vi "Main_TestStand_v2.vi"() -> ()   [LabVIEW 2019]
uses:
  <vilib>/Platform/TimedLoop/XDataNode/timing_clust.ctl
  <vilib>/Platform/TimedLoop/XDataNode/nitl_modes.ctl
  <vilib>/Platform/TimedLoop/XDataNode/wakeup.ctl
  <vilib>/platform/TimedLoop/XDataNode/XDataNode.xnode
  <vilib>/ptbypt/NI_PtbyPt.lvlib
  <vilib>/Platform/TimedLoop/XDataNode/XDNodeRunTimeDep.lvlib
panel:
  out "motor signal":cluster{dbl, dbl}
  out "raw x axis imu data":i16
  out "motor 1 correction":dbl(graph)
  out "Labview PID Inputs (should not match gains) 2":T1
  in  "Proportional Gain (Kc) 2":dbl
  in  "Derivative Gain (Kd) 2":dbl format="%#_13g"
  in  "Integral Gain (Ki) 2":dbl format="%#_13g"
  out "Raw x value":dbl(graph)
  in  "Adjustment x":dbl format="%0.2f"
  in  "low cutoff freq x":dbl=0.01 format="%#_13g"
  out "Filtered Correction x":dbl format="%0.2f"
  out "Filtered Correction x":dbl(graph)
  out "Motor 2 Correction":dbl
  out "Motor 1 Correction":dbl
  out "error out":errorcluster
  out "error out 2":errorcluster
  out "error out 6":errorcluster
  in  "Initial Motor Power":dbl
  in  "Stop":bool
  # "X-Axis Gains"
  # "Y-Axis Gains"
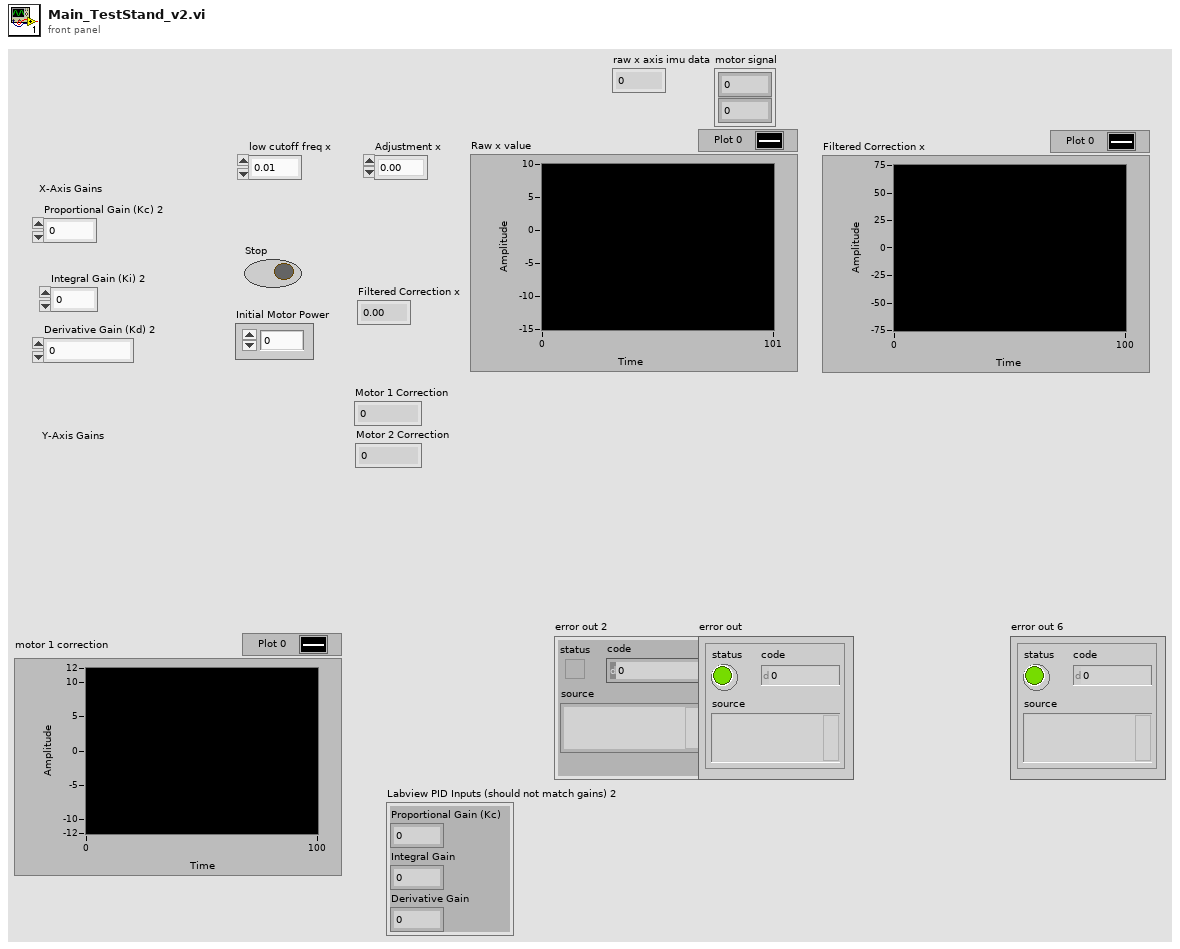
[diagram p1: front panel]
types:
  T1 = cluster{"Proportional Gain (Kc)":dbl, "Integral Gain":dbl, "Derivative Gain":dbl}
  T2 = typedef "XDNodeRunTimeDep.lvlib/timing_clust.ctl" = cluster{"Expected End [f-1]":u64, "Actual End [f-1]":u64, "Finished Late? [f-1]":bool, "Expected End [i-1]":u64, "Actual End [i-1]":u64, "Finished Late? [i-1]":bool, "Expected Start [i]":u64, "Actual Start [i]":u64, "Expected Start [f]":u64, "Actual Start [f]":u64, "Source Name":string, "Structure Name":string, "Period":i64, "Deadline":i64, "Offset":i64, "Start":i64, "Priority":i32, "Timeout":i32, "Mode":T3, "Wakeup Reason":T4, "Error":errorcluster, "Source Type":string, "Secondary Source Type":string, "Global End Time":u64, "Global Start Time":u64, "Frame Duration":u64, "Iteration Duration":u64, "Assigned CPU":i32, "I/O Scan Engine Mode":u32}
  T3 = typedef "XDNodeRunTimeDep.lvlib/nitl_modes.ctl" = enum32{"No Change", "Process missed periods, maintain original phase", "Discard missed periods, maintain original phase", "Process missed periods, ignore original phase", "Discard missed periods, ignore original phase"}
  T4 = typedef "XDNodeRunTimeDep.lvlib/wakeup.ctl" = enum32{"Normal", "Aborted", "Asynchronous wakeup", "Timing source error", "Timed loop error", "Timeout"}
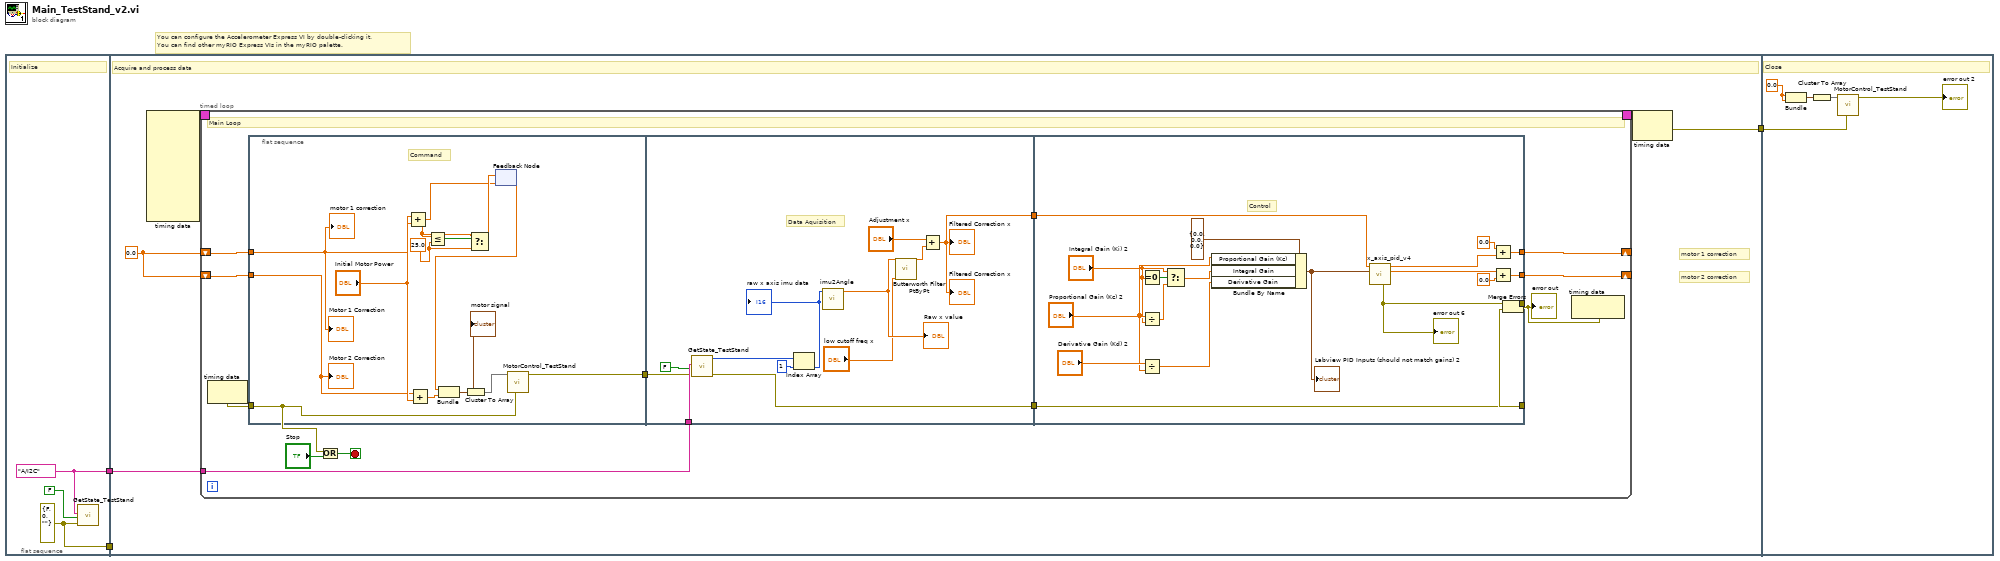
[diagram p0: block diagram]
diagram:
  # "You can configure the Accelerometer Express VI by double-clicking it.\nYou can find other myRIO Express VIs in the myRIO palette."
  n1 = flat-sequence {
    tunnel: [w6] -> w3
    tunnel: [w4] -> w2
    tunnel: [w7] -> w1
    tunnel: w3 -> [w11]
    tunnel: w2 -> [_]
    tunnel: w1 -> [w78]
    frame #0 {
      w6 = tag "A/I2C" ("IMU Channel")
      w4 = errorcluster {"status"=FALSE, "code"=0, "source"=""} ("error in (no error)")
      # "Initialize"
      n2 = call "GetState_TestStand.vi"("error in (no error)"=w4, "Calibrate?"=FALSE, "IMU Channel"=w6) -> ()  [unwired: 4 in, 3 out]
    }
    frame #1 {
      w8 = 0.0
      # "motor 2 correction"
      # "motor 1 correction"
      # "Acquire and process data"
      n3 = node-c288() -> (w10:T2)  [unwired: 9 in]
      n4 = timed-loop {
        tunnel: w11 -> [w22]
        timing: w10 -> [_]
        timing-out: [_] -> w9
        shift-right: [w19] -> _
        shift-left: w8 -> [w17]
        shift-right: [w18] -> _
        shift-left: w8 -> [w16]
        stop <- w25 stop-if-true
        # "Main Loop"
        n5 = node-c288() -> (w12:errorcluster)  [unwired: 1 in]
        n6 = flat-sequence {
          tunnel: w17 -> [w31]
          tunnel: w16 -> [w34]
          tunnel: w12 -> [w33]
          tunnel: [w32] -> w15
          tunnel: w22 -> [w50]
          tunnel: [w41] -> w21
          tunnel: w15 -> [w40]
          tunnel: [w39] -> w14
          tunnel: [w59] -> w23
          tunnel: w21 -> [w58]
          tunnel: [w55] -> w19
          tunnel: [w54] -> w18
          tunnel: w14 -> [w51]
          tunnel: [w51] -> w13
          frame #0 {
            w27 = 25.0 ("y")
            # "Command"
            n7 = Add(x=w31, y="Initial Motor Power") -> (x+y=w26:dbl)
            n8 = Add(x=w34, y="Initial Motor Power") -> (x+y=w38:dbl)
            n9 = Less Or Equal?(x=w26, y=w27) -> (x <= y?=w28:bool)
            n10 = Select(t=w26, s=w28, f=w27) -> (s? t:f=w30:dbl)
            n11 = feedback-in #1(w30) -> ()
            n12 = feedback #1(w26) -> (w29:dbl)
            n13 = Bundle(w29, w38) -> (w36:cluster{dbl, dbl})  [unwired: 1 in]
            "motor signal" <- w36
            n14 = Cluster To Array(cluster=w36) -> (array=w35:dbl[])
            n15 = call "MotorControl_TestStand.vi"("error in (no error)"=w33, "Array"=w35) -> ("error out"=w32:errorcluster)  [unwired: 9 in]
            "Motor 1 Correction" <- w31
            "Motor 2 Correction" <- w34
            "motor 1 correction" <- w31
          }
          frame #1 {
            # "Data Aquisition"
            n16 = call "GetState_TestStand.vi"("error in (no error)"=w40, "Calibrate?"=FALSE, "IMU Channel"=w50) -> ("error out"=w39:errorcluster, "imu accel"=w43:i16[])  [unwired: 4 in, 1 out]
            n17 = Index Array(array=w43, index=1) -> (element=w42:i16)
            "raw x axis imu data" <- w42
            n18 = call "imu2Angle.vi"("Sensor Input"=w42) -> ("Angle (radians)"=w48:dbl)  [unwired: 10 in]
            "Raw x value" <- w48
            n19 = call <vilib>:"Butterworth Filter PtByPt.vi"("low cutoff freq: fl"="low cutoff freq x", "x"=w48) -> ("Filtered x"=w46:dbl)  [unwired: 7 in, 1 out]
            n20 = Add(x="Adjustment x", y=w46) -> (x+y=w41:dbl)
            "Filtered Correction x" <- w41
            "Filtered Correction x" <- w41
          }
          frame #2 {
            # "Control"
            n21 = Equal To 0?(x="Integral Gain (Ki) 2") -> (x = 0?=w64:bool)
            n22 = Divide(x="Proportional Gain (Kc) 2", y="Integral Gain (Ki) 2") -> (x/y=w62:dbl)
            n23 = Divide(x="Derivative Gain (Kd) 2", y="Proportional Gain (Kc) 2") -> (x/y=w66:dbl)
            n24 = Select(t="Integral Gain (Ki) 2", s=w64, f=w62) -> (s? t:f=w61:dbl)
            n25 = Bundle By Name(cluster=T1 {"Proportional Gain (Kc)"=0.0, "Integral Gain"=0.0, "Derivative Gain"=0.0} ("PID Gains (x-axis)"), "Proportional Gain (Kc)"="Proportional Gain (Kc) 2", "Integral Gain"=w61, "Derivative Gain"=w66) -> (w60:T1)
            "Labview PID Inputs (should not match gains) 2" <- w60
            n26 = call "x_axis_pid_v4.vi"("PID Gains"=w60, "X In"=w58) -> ("Motor 2"=w56:dbl, "Motor 1"=w57:dbl, "error out"=w59:errorcluster)  [unwired: 5 in, 2 out]
            "error out 6" <- w59
            n27 = Add(x=0.0, y=w57) -> (x+y=w55:dbl)
            n28 = Add(x=w56, y=0.0) -> (x+y=w54:dbl)
          }
        }
        n29 = Or(x=w12, y="Stop") -> (x .or. y?=w25:bool)
        n30 = Merge Errors(w23, w13) -> (w20:errorcluster)
        "error out" <- w20
        n31 = node-c288(w20) -> ()  [unwired: 1 out]
      }
      n32 = node-c288(w9) -> (w7:errorcluster)
    }
    frame #2 {
      w81 = 0.0
      # "Close"
      n33 = Bundle(w81, w81) -> (w80:cluster{dbl, dbl})  [unwired: 1 in]
      n34 = Cluster To Array(cluster=w80) -> (array=w79:dbl[])
      n35 = call "MotorControl_TestStand.vi"("error in (no error)"=w78, "Array"=w79) -> ("error out"=→"error out 2":errorcluster)  [unwired: 9 in]
    }
  }
